vi "Main.vi"(0 "Left Buttons":T4, 1 "User Input":string, 5 "Right Buttons":T3, 7 "Card Simulator":bool, 9 "Enter":bool, 11 "Error in":errorcluster) -> (4 "Right Menu":T1, 6 "Left Menu":T2, 8 "ATM Messages":string, 15 "Error out":errorcluster)   [LabVIEW 2020, in "Automated teller machine.lvlib"]
doc: "This machine replicates the working of a automated teller machine and this can be used to deposit and get money with the right credentials."
uses:
  Automated teller machine.lvlib
  Typedefs/Queue driver operations.ctl
  Typedefs/Left menu.ctl
  Typedefs/Right menu.ctl
  Typedefs/Left buttons.ctl
  Typedefs/Right buttons.ctl
  Typedefs/Data Cluster.ctl
  Typedefs/variant data.ctl
panel:
  out "Previous time":dbl
  # "AUTOMATED TELLER MACHINE"
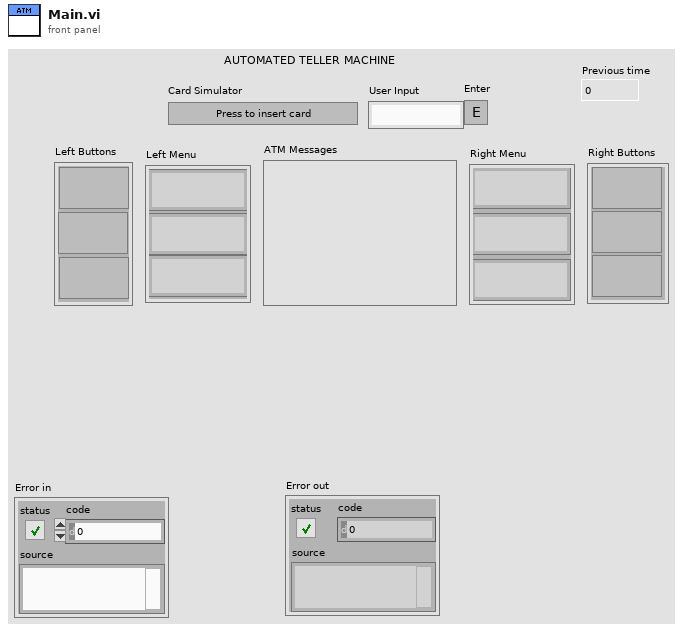
[diagram p1: front panel]
types:
  T1 = cluster{"R1 Menu":string, "R2 Menu":string, "R3 Menu":string}
  T2 = cluster{"L1 Menu":string, "L2 Menu":string, "L3 Menu":string}
  T3 = cluster{"Deposit ":bool, "Withdraw ":bool, "Fast Cash $50 ":bool}
  T4 = cluster{"None ":bool, "Balance Inquiry ":bool, "Return card & Terminate ":bool}
  T5 = typedef "variant data.ctl" = cluster{"State":string, "Data":variant}
  T6 = typedef "Automated teller machine.lvlib/Data Cluster.ctl" = cluster{"Left Menu":T7, "Right Menu":T8, "ATM Messages":string, "Account number":i32, "Card Simulator":bool, "Enter":bool, "Left buttons":T9, "Right buttons":T10, "Path":path, "Timing":cluster{"Start time":dbl, "Elapsed time":dbl, "Previous time":dbl, "Started":bool, "Paused":bool}, "Enable controls":refnum<vi>[], "Disable controls":refnum<vi>[], "User enter":refnum<vi>[], "Left menu":refnum<vi>[], "Right menu":refnum<vi>[], "Left button":refnum<vi>[], "Right button":refnum<vi>[]}
  T7 = typedef "Automated teller machine.lvlib/Left menu.ctl" = cluster{"L1 menu":string, "L2 menu":string, "L3 menu":string}
  T8 = typedef "Automated teller machine.lvlib/Right menu.ctl" = cluster{"R1 menu":string, "R2 menu":string, "R3 menu":string}
  T9 = typedef "Automated teller machine.lvlib/Left buttons.ctl" = cluster{"L1":bool, "L2":bool, "L3":bool}
  T10 = typedef "Automated teller machine.lvlib/Right buttons.ctl" = cluster{"R1":bool, "R2":bool, "R3":bool}
  T11 = typedef "Automated teller machine.lvlib/Queue driver operations.ctl" = enum16{"Create Q", "Enqueue", "Enstack", "Dequeue", "Flush", "Release"}
  T12 = cluster{"Start time":dbl, "Elapsed time":dbl, "Previous time":dbl, "Started":bool, "Paused":bool}
  T13 = enum8{"Enabled", "Disabled", "Disabled and Grayed Out"}
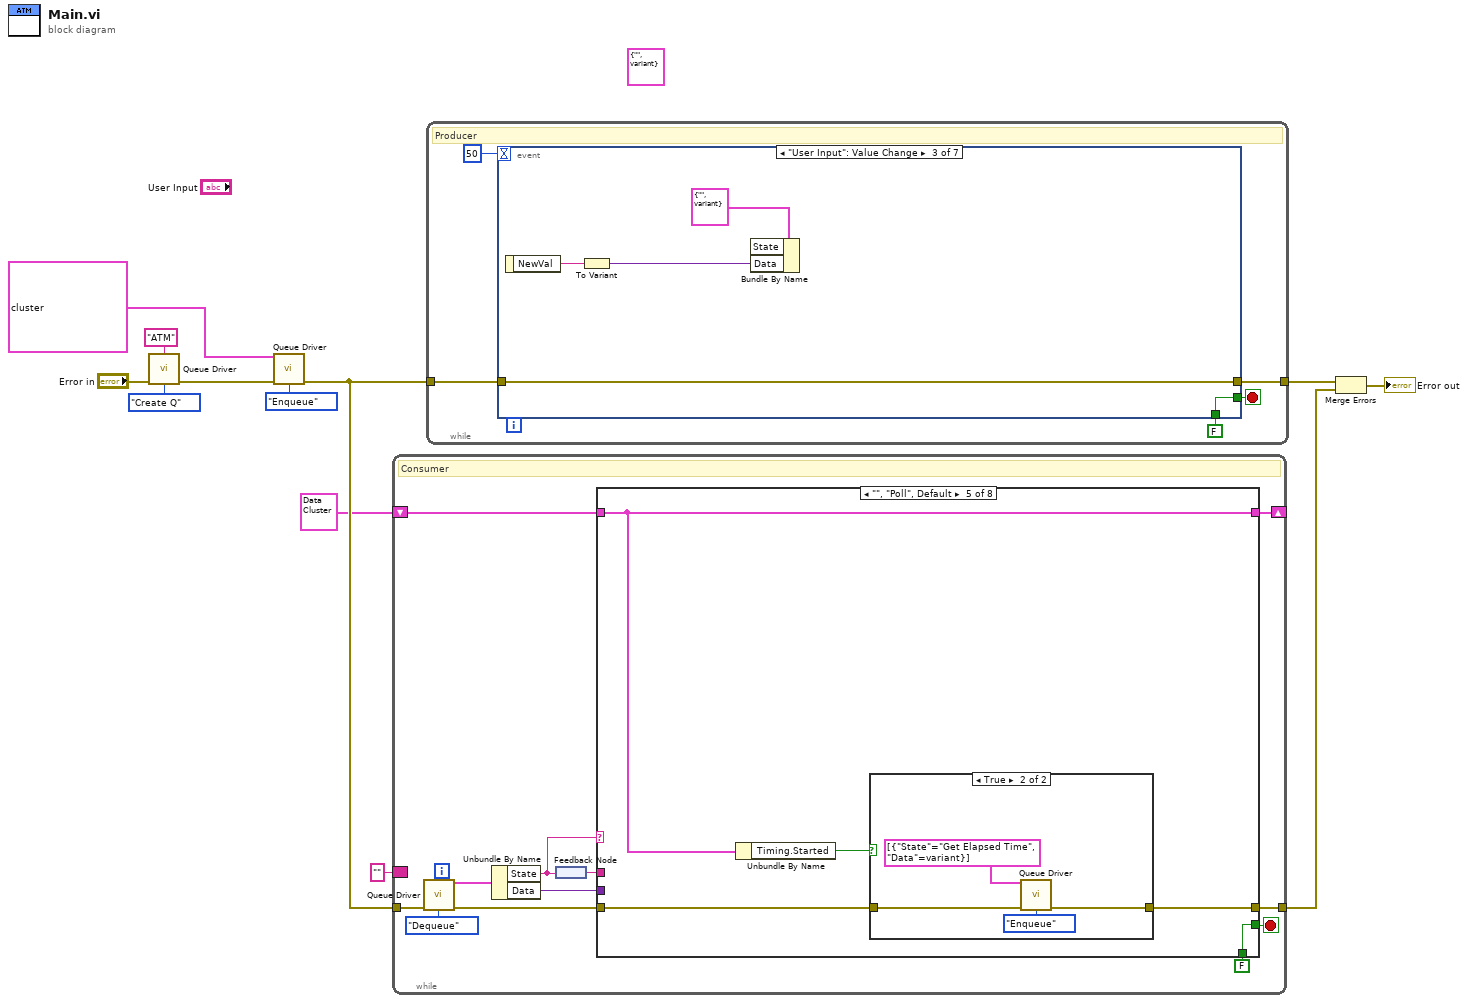
[diagram p0: block diagram]
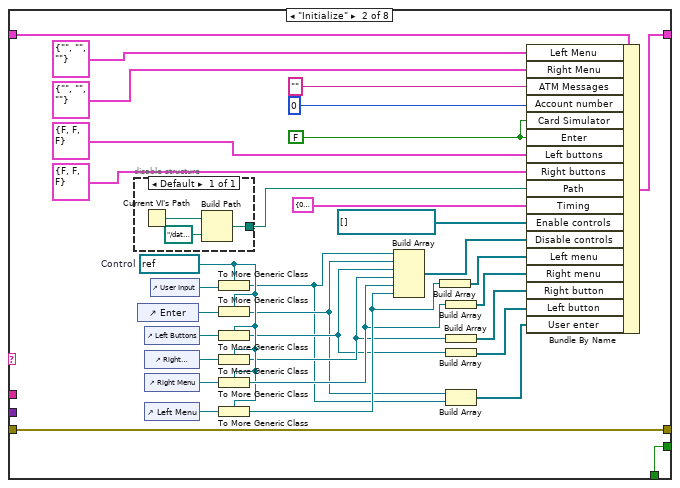
[diagram p3: hidden frame]
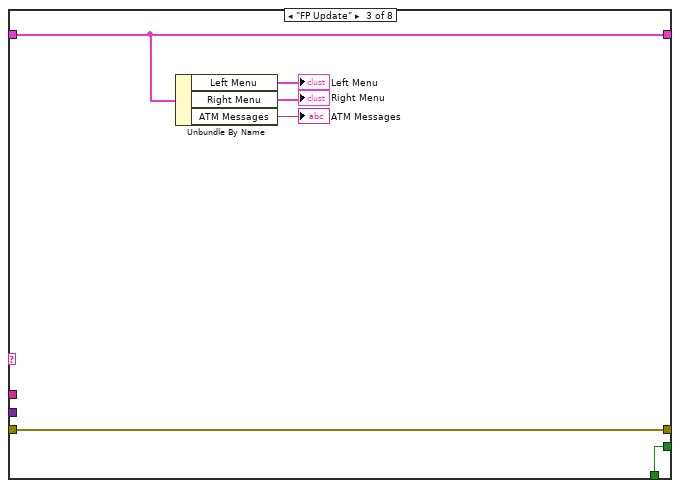
[diagram p4: hidden frame]
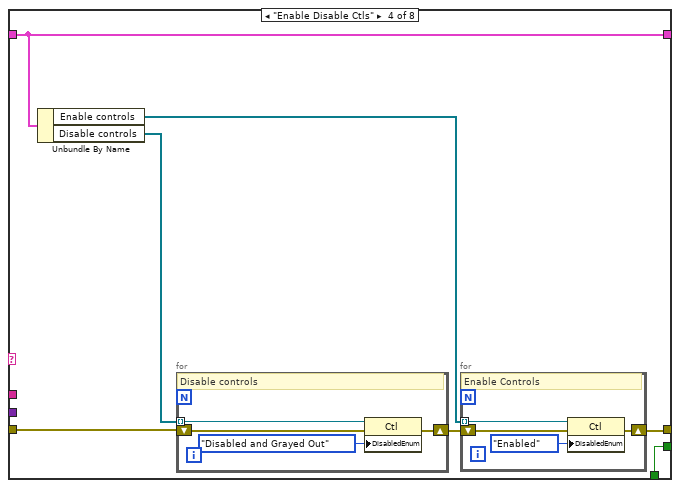
[diagram p5: hidden frame]
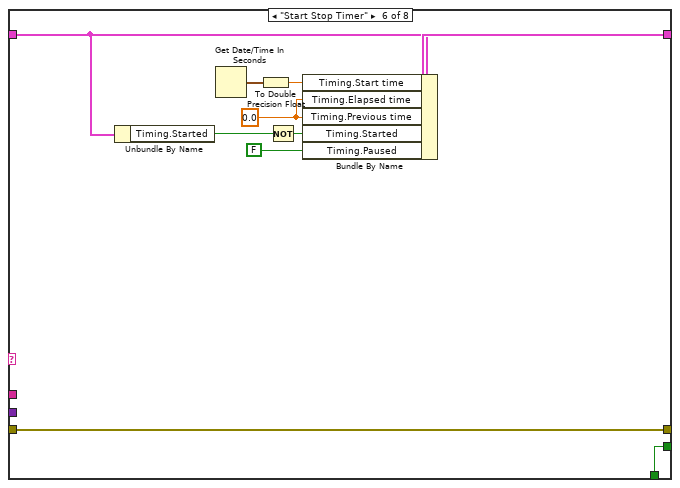
[diagram p7: hidden frame]
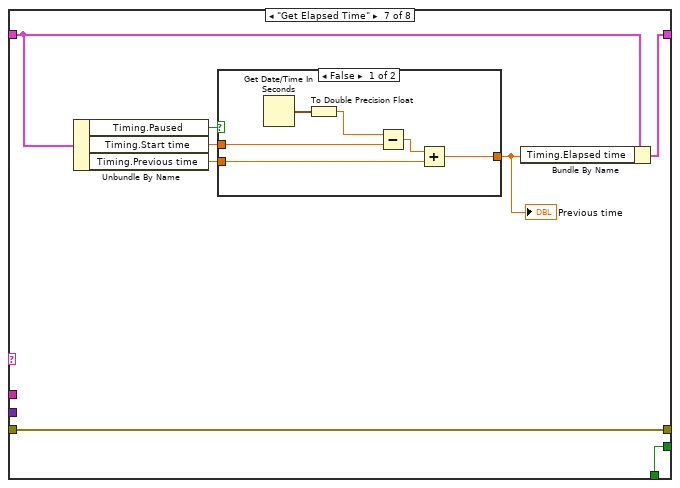
[diagram p8: hidden frame]
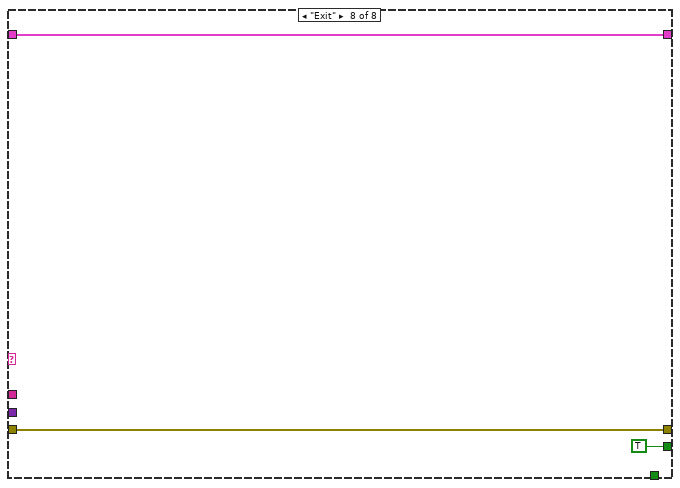
[diagram p10: hidden frame]
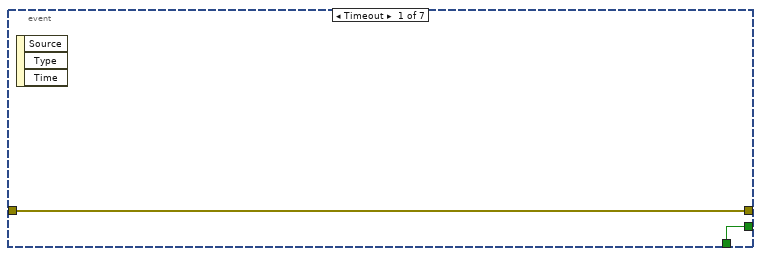
[diagram p11: hidden frame]
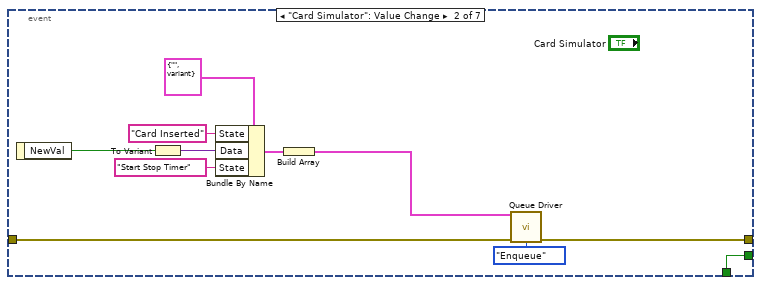
[diagram p12: hidden frame]
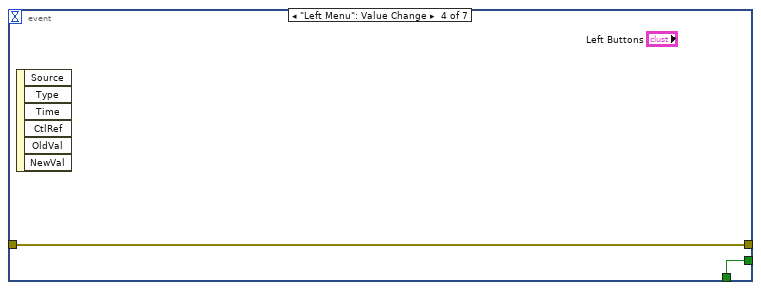
[diagram p13: hidden frame]
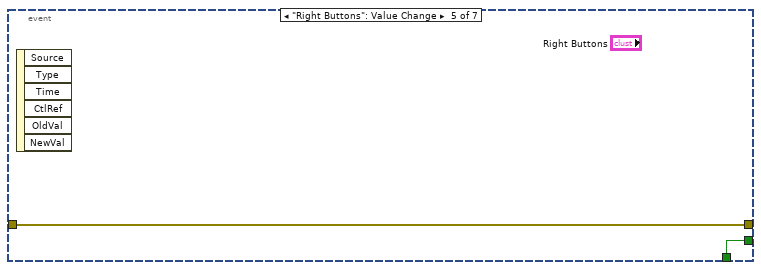
[diagram p14: hidden frame]
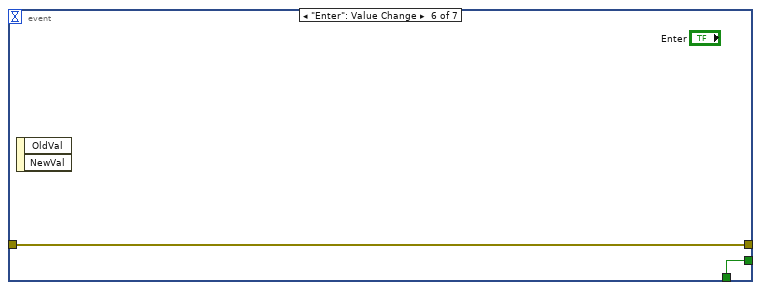
[diagram p15: hidden frame]
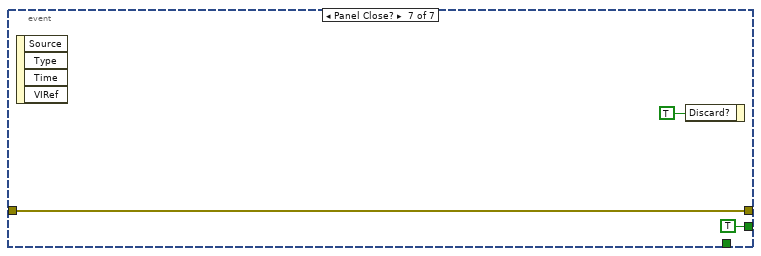
[diagram p16: hidden frame]
diagram:
  (unwired) T5 {"State"="", "Data"=variant} ("Dequeue data")
  n1 = call "Queue Driver.vi"("Name"="ATM", "Error in"="Error in", "Queue operations"=Queue_driver_operations."Create Q") -> ("Error out"=w9:errorcluster)  [unwired: 11 in, 1 out]
  n2 = call "Queue Driver.vi"("States and data"=cluster{"State":string, "Data":variant}[] [{"State"="Initialize", "Data"=variant}, {"State"="FP Update", "Data"=variant}], "Error in"=w9, "Queue operations"=Queue_driver_operations."Enqueue") -> ("Error out"=w5:errorcluster)  [unwired: 11 in, 1 out]
  n3 = while {
    border: "" ("State") -> [_]
    tunnel: w5 -> [w20]
    tunnel: [w17] -> w3
    shift-right: [w13] -> _
    shift-left: T6 {"Left Menu"={"L1 menu"="", "L2 menu"="", "L3 menu"=""}, "Right Menu"={"R1 menu"="", "R2 menu"="", "R3 menu"=""}, "ATM Messages"="", "Account number"=0, "Card Simulator"=FALSE, "Enter"=FALSE, "Left buttons"={"L1"=FALSE, "L2"=FALSE, "L3"=FALSE}, "Right buttons"={"R1"=FALSE, "R2"=FALSE, "R3"=FALSE}, "Path"=path "", "Timing"={"Start time"=0.0, "Elapsed time"=0.0, "Previous time"=0.0, "Started"=FALSE, "Paused"=FALSE}, "Enable controls"=[], "Disable controls"=[], "User enter"=[], "Left menu"=[], "Right menu"=[], "Left button"=[], "Right button"=[]} -> [w14]
    stop <- w16 stop-if-true
    # "Consumer"
    n4 = call "Queue Driver.vi"("Error in"=w20, "Queue operations"=Queue_driver_operations."Dequeue") -> ("Dequeue data"=w22:cluster{"State":string, "Data":variant}, "Error out"=w19:errorcluster)  [unwired: 12 in]
    n5 = Unbundle By Name(w22) -> ("State"=w18:string, "Data"=w21:variant)
    n6 = feedback-in #1(w18) -> ()
    n7 = feedback #1() -> (w24:string)
    n8 = case shown="\"\", \"Poll\", Default" w18 {
      tunnel: w24 -> [_ _ _ _ _ _ _ _]
      tunnel: w21 -> [_ _ _ _ _ _ _ _]
      tunnel: w19 -> [w26 w60 w69 w74 w86 w104 w112 w121]
      tunnel: [w26 w60 w69 w73 w85 w104 w112 w121] -> w17
      tunnel: [w27 w59 w68 w76 w89 w103 w111 TRUE] -> w16
      tunnel: FALSE -> [w27 w59 w68 w76 w89 w103 w111 _]
      tunnel: w14 -> [w25 w58 w67 w72 w88 w99 w107 w120]
      tunnel: [w25 w57 w67 w72 w88 w102 w106 w120] -> w13
      frame "Get ref" {
      }
      frame "Initialize" {
        w37 = refnum<vi> refnum  # Control
        w51 = FALSE ("Enter")
        n9 = disable-structure shown="Default" {
          disable-tunnel: [w61] -> w49
          frame Enabled {
            n10 = Current VI's Path() -> (path=w63:path)
            n11 = Build Path(base path=w63, name or relative path=path "../data/Accounts.txt") -> (appended path=w61:path)
          }
        }
        n12 = control-ref of="Enter"() -> (w34:refnum<vi>)
        n13 = control-ref of="Left Buttons"() -> (w33:refnum<vi>)
        n14 = control-ref of="Right Buttons"() -> (w45:refnum<vi>)
        n15 = control-ref of="Right Menu"() -> (w44:refnum<vi>)
        n16 = control-ref of="Left Menu"() -> (w43:refnum<vi>)
        n17 = control-ref of="User Input"() -> (w46:refnum<vi>)
        n18 = To More Generic Class(target class=w37, reference=w46) -> (generic class reference=w29:refnum<vi>)
        n19 = To More Generic Class(target class=w37, reference=w34) -> (generic class reference=w30:refnum<vi>)
        n20 = To More Generic Class(target class=w37, reference=w33) -> (generic class reference=w32:refnum<vi>)
        n21 = To More Generic Class(target class=w37, reference=w45) -> (generic class reference=w36:refnum<vi>)
        n22 = To More Generic Class(target class=w37, reference=w44) -> (generic class reference=w39:refnum<vi>)
        n23 = To More Generic Class(target class=w37, reference=w43) -> (generic class reference=w40:refnum<vi>)
        n24 = Build Array(w29, w30, w32, w36, w39, w40) -> (w42:refnum<vi>[])
        n25 = Build Array(w40) -> (w41:refnum<vi>[])
        n26 = Build Array(w39) -> (w38:refnum<vi>[])
        n27 = Build Array(w36) -> (w35:refnum<vi>[])
        n28 = Build Array(w32) -> (w31:refnum<vi>[])
        n29 = Build Array(w30, w29) -> (w28:refnum<vi>[])
        n30 = Bundle By Name(cluster=w58, "Left Menu"=T7 {"L1 menu"="", "L2 menu"="", "L3 menu"=""}, "Right Menu"=T8 {"R1 menu"="", "R2 menu"="", "R3 menu"=""}, "ATM Messages"="", "Account number"=0, "Card Simulator"=w51, "Enter"=w51, "Left buttons"=T9 {"L1"=FALSE, "L2"=FALSE, "L3"=FALSE}, "Right buttons"=T10 {"R1"=FALSE, "R2"=FALSE, "R3"=FALSE}, "Path"=w49, "Timing"=T12 {"Start time"=0.0, "Elapsed time"=0.0, "Previous time"=0.0, "Started"=FALSE, "Paused"=FALSE}, "Enable controls"=refnum<vi>[] [], "Disable controls"=w42, "Left menu"=w41, "Right menu"=w38, "Right button"=w35, "Left button"=w31, "User enter"=w28) -> (w57:T6)
      }
      frame "FP Update" {
        n31 = Unbundle By Name(w67) -> ("Left Menu"=→"Left Menu":T7, "Right Menu"=→"Right Menu":T8, "ATM Messages"=→"ATM Messages":string)
      }
      frame "Enable Disable Ctls" {
        n32 = Unbundle By Name(w72) -> ("Enable controls"=w71:refnum<vi>[], "Disable controls"=w70:refnum<vi>[])
        n33 = for {
          shift-right: [w83] -> w75
          shift-left: w74 -> [w84]
          tunnel: w70 -> [w81] mode=indexing
          # "Disable controls"
          n34 = property class="Ctl"(reference=w81, error in=w84, "DisabledEnum"=T13."Disabled and Grayed Out" ("Disabled")) -> (error out=w83:errorcluster)  [unwired: 1 out]
        }
        n35 = for {
          shift-right: [w79] -> w73
          shift-left: w75 -> [w80]
          tunnel: w71 -> [w77] mode=indexing
          # "Enable Controls"
          n36 = property class="Ctl"(reference=w77, error in=w80, "DisabledEnum"=T13."Enabled" ("Disabled")) -> (error out=w79:errorcluster)  [unwired: 1 out]
        }
      }
      frame "", "Poll", Default {
        n37 = Unbundle By Name(w88) -> ("Timing.Started"=w87:bool)
        n38 = case shown="True" w87 {
          tunnel: w86 -> [w90 w93]
          tunnel: [w90 w92] -> w85
          frame False {
          }
          frame True {
            n39 = call "Queue Driver.vi"("States and data"=cluster{"State":string, "Data":variant}[] [{"State"="Get Elapsed Time", "Data"=variant}], "Error in"=w93, "Queue operations"=Queue_driver_operations."Enqueue") -> ("Error out"=w92:errorcluster)  [unwired: 11 in, 1 out]
          }
        }
      }
      frame "Start Stop Timer" {
        w98 = 0.0 ("Timing.Elapsed time")
        n40 = Unbundle By Name(w99) -> ("Timing.Started"=w96:bool)
        n41 = Get Date/Time In Seconds() -> (seconds since 1Jan1904=w101:timestamp)
        n42 = To Double Precision Float(number=w101) -> (double precision float=w100:dbl)
        n43 = Not(x=w96) -> (.not. x?=w97:bool)
        n44 = Bundle By Name(cluster=w99, "Timing.Start time"=w100, "Timing.Elapsed time"=w98, "Timing.Previous time"=w98, "Timing.Started"=w97, "Timing.Paused"=FALSE) -> (w102:T6)
      }
      frame "Get Elapsed Time" {
        n45 = Unbundle By Name(w107) -> ("Timing.Paused"=w110:bool, "Timing.Start time"=w109:dbl, "Timing.Previous time"=w108:dbl)
        n46 = case shown="False" w110 {
          tunnel: w109 -> [w115 _]
          tunnel: w108 -> [w114 w119]
          tunnel: [w113 w119] -> w105
          frame False {
            n47 = Get Date/Time In Seconds() -> (seconds since 1Jan1904=w118:timestamp)
            n48 = To Double Precision Float(number=w118) -> (double precision float=w117:dbl)
            n49 = Subtract(x=w117, y=w115) -> (x-y=w116:dbl)
            n50 = Add(x=w116, y=w114) -> (x+y=w113:dbl)
          }
          frame True {
          }
        }
        "Previous time" <- w105
        n51 = Bundle By Name(cluster=w107, "Timing.Elapsed time"=w105) -> (w106:T6)
      }
      frame "Exit" {
      }
    }
  }
  n52 = while {
    tunnel: w5 -> [w126]
    tunnel: [w125] -> w4
    stop <- w124 stop-if-true
    # "Producer"
    n53 = event shown="[2] \"User Input\": Value Change" {
      selector: _ -> [_ _ _ _ _ _ _]
      dyn-events: _ -> [_ _ _ _ _ _ _]
      timeout: 50 -> [_ _ _ _ _ _ _]
      tunnel: w126 -> [w128 w132 w145 w146 w148 w151 w152]
      tunnel: [w128 w131 w145 w146 w148 w151 w152] -> w125
      tunnel: [w129 w140 w144 w147 w149 w150 TRUE] -> w124
      tunnel: FALSE -> [w129 w140 w144 w147 w149 w150 _]
      event Timeout {
        n54 = event-data() -> ()  [unwired: 1 in, 3 out]
      }
      event "Card Simulator": Value Change {
        n55 = event-data() -> ("NewVal"=w139:bool)  [unwired: 1 in]
        n56 = To Variant(anything=w139) -> (Variant=w137:variant)
        n57 = Bundle By Name(cluster=T5 {"State"="", "Data"=variant} ("Dequeue data"), "State"="Card Inserted", "Data"=w137, "State"="Start Stop Timer") -> (w134:T5)
        n58 = Build Array(w134) -> (w130:T5[])
        n59 = call "Queue Driver.vi"("States and data"=w130, "Error in"=w132, "Queue operations"=Queue_driver_operations."Enqueue") -> ("Error out"=w131:errorcluster)  [unwired: 11 in, 1 out]
      }
      event "User Input": Value Change {
        n60 = event-data() -> ("NewVal"=w143:string)  [unwired: 1 in]
        n61 = To Variant(anything=w143) -> (Variant=w141:variant)
        n62 = Bundle By Name(cluster=T5 {"State"="", "Data"=variant} ("Dequeue data"), "Data"=w141) -> ()  [unwired: 1 in, 1 out]
      }
      event "Left Menu": Value Change {
        n63 = event-data() -> ()  [unwired: 1 in, 6 out]
      }
      event "Right Buttons": Value Change {
        n64 = event-data() -> ()  [unwired: 1 in, 6 out]
      }
      event "Enter": Value Change {
        n65 = event-data() -> ()  [unwired: 1 in, 2 out]
      }
      event Panel Close? {
        n66 = event-data() -> ()  [unwired: 1 in, 4 out]
        n67 = event-data("Discard?"=TRUE) -> ()  [unwired: 1 in, 1 out]
      }
    }
  }
  n68 = Merge Errors(w4, w3) -> (→"Error out":errorcluster)
